vi "Init Load Cell DaqChannel.vi"(0 "task in":refnum<k21>, 1 "LoadCellParams":T2={"Excitation Value (Volts)"=2.5, "mV/V"=2.0, "Max Weight (lbs)"=500.0}, 2 "Do Offset Null?":bool, 5 "Physical Channels":tag, 7 "number samples":i32=1000, 9 "Rate":dbl=25000.0, 11 "error in (no error)":errorcluster, 12 "ShuntCalParams":T1={"Load Cell bridge resistance (Ohms)"=120.0, "9237 Internal shunt resistance (Ohms)"=100000.0, "shunt element location"=14813} {"shunt element location" items=["R1"=12465, "R2"=12466, "R3"=12467, "R4"=14813, "None"=10230]; "9237 Internal shunt resistance (Ohms)" format="%#.3p"}, 13 "Do Shunt Cal?":bool) -> (4 "task out":refnum<k21>, 15 "error out":errorcluster)   [LabVIEW 2017]
uses:
  <vilib>/DAQmx/create/scale.llb/DAQmx Create Scale (Linear).vi
  <vilib>/DAQmx/create/channels.llb/DAQmx Create Channel (AI-Voltage-Custom with Excitation).vi
  <vilib>/DAQmx/configure/timing.llb/DAQmx Timing (Sample Clock).vi
  <userlib>/_OpenG.lib/error/error.llb/Filter Error Codes (Array)__ogtk.vi
  <vilib>/DAQmx/calibration/calibrationInfo.llb/DAQmx Perform Shunt Calibration Ex (Bridge).vi
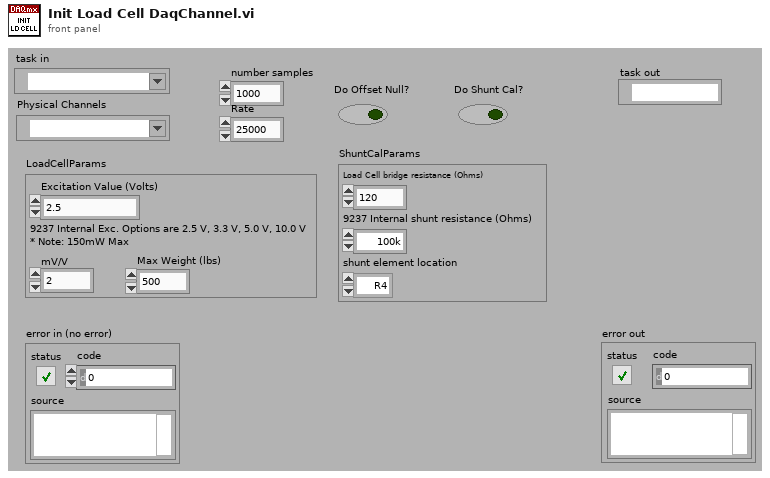
[diagram p1: front panel]
types:
  T1 = cluster{"Load Cell bridge resistance (Ohms)":dbl, "9237 Internal shunt resistance (Ohms)":dbl, "shunt element location":i32}
  T2 = cluster{"Excitation Value (Volts)":dbl, "mV/V":dbl, "Max Weight (lbs)":dbl}
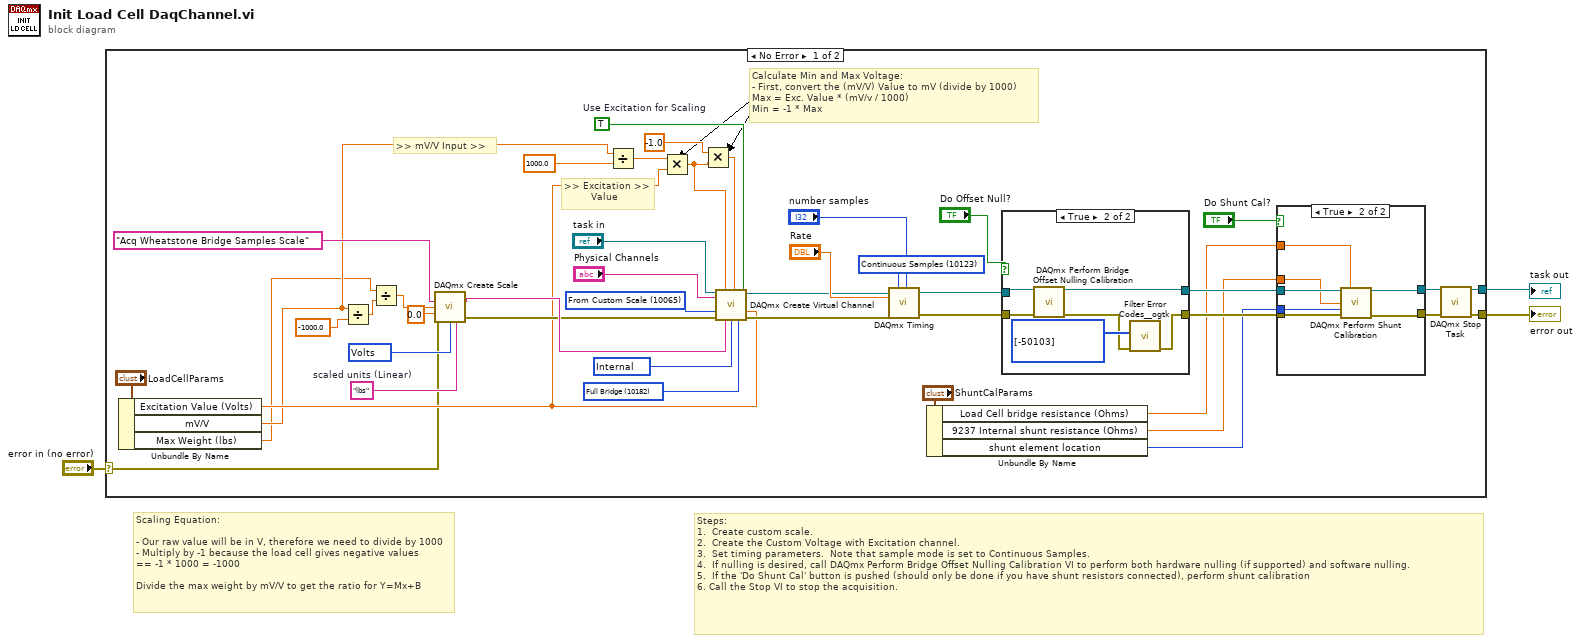
[diagram p0: block diagram]
diagram:
  # "Scaling Equation:\n\n- Our raw value will be in V, therefore we need to divide by 1000\n- Multiply by -1 because the load cell gives negative values\n== -1 * 1000 = -1000\n\nDivide the max weight by mV/V to get the ratio for Y=Mx+B"
  # "Steps:\n1.  Create custom scale.\n2.  Create the Custom Voltage with Excitation channel.\n3.  Set timing parameters.  Note that sample mode is set to Continuous Samples.\n4.  If nulling is desired, call DAQmx Perform Bridge Offset Nulling Calibration VI to perform both hardware nulling (if supported) and software nulling.\n5.  If the 'Do Shunt Cal' button is pushed (should only be done if you have shunt resistors connected), perform shunt calibration \n6. Call the Stop VI to stop the acquisition."
  n1 = case shown="No Error" "error in (no error)" {
    selector: "error in (no error)" -> [w5 w65]
    tunnel: [w18 w65] -> w3
    tunnel: [w16 _] -> w2
    frame No Error {
      w33 = "lbs"  # scaled units (Linear)
      w29 = 10348 items=["Volts"=10348, "Amps"=10342, "Deg F"=10144, "Deg C"=10143, "Deg R"=10145, "Kelvins"=10325, "Strain"=10299, "Ohms"=10384, "Hz"=10373, "Seconds"=10364] ("pre-scaled units")
      w36 = 10200 items=["Internal"=10200, "External"=10167, "None"=10230] ("Excitation Source")
      w35 = 10182 items=["Full Bridge"=10182, "Half Bridge"=10187, "Quarter Bridge"=10270, "No Bridge"=10228] ("Bridge Configuration")
      w30 = TRUE  # Use Excitation for Scaling
      w37 = 10065 items=["Volts"=10348, "From Custom Scale"=10065] ("units")
      w47 = 10123 items=["Finite Samples"=10178, "Continuous Samples"=10123] ("sample mode")
      # ">> Excitation >>\n         Value"
      # ">> mV/V Input >>"
      # "Calculate Min and Max Voltage:\n- First, convert the (mV/V) Value to mV (divide by 1000)\nMax = Exc. Value * (mV/v / 1000)\nMin = -1 * Max"
      n2 = Unbundle By Name("LoadCellParams") -> ("Excitation Value (Volts)"=w13:dbl, "mV/V"=w12:dbl, "Max Weight (lbs)"=w11:dbl)
      n3 = Divide(x=w12, y=-1000.0) -> (x/y=w23:dbl)
      n4 = Divide(x=w11, y=w23) -> (x/y=w20:dbl)
      n5 = call-poly <vilib>:"DAQmx Create Scale.vi"("name"="Acq Wheatstone Bridge Samples Scale", "slope"=w20, "y-intercept"=0.0 ("B"), "error in"=w5, "pre-scaled units"=w29, "scaled units"=w33) -> ("scale out"=w40:tag, "error out"=w39:errorcluster)  [unwired: 8 in]
      n6 = Divide(x=w12, y=1000.0) -> (x/y=w25:dbl)
      n7 = Multiply(x=w25, y=w13) -> (x*y=w22:dbl)
      n8 = Multiply(x=-1.0, y=w22) -> (x*y=w21:dbl)
      n9 = call-poly <vilib>:"DAQmx Create Virtual Channel.vi"("task in"="task in", "maximum value"=w22, "minimum value"=w21, "physical channels"="Physical Channels", "use excitation for scaling"=w30, "units"=w37, "voltage excitation value"=w13, "error in"=w39, "custom scale name"=w40, "voltage excitation source"=w36, "bridge configuration"=w35) -> ("task out"=w32:refnum<k21>, "error out"=w31:errorcluster)  [unwired: 3 in]
      n10 = call-poly <vilib>:"DAQmx Timing.vi"("task/channels in"=w32, "sample mode"=w47, "samples per channel"="number samples", "rate"="Rate", "error in"=w31) -> ("task out"=w42:refnum<k21>, "error out"=w41:errorcluster)  [unwired: 9 in]
      n11 = Unbundle By Name("ShuntCalParams") -> ("Load Cell bridge resistance (Ohms)"=w8:dbl, "9237 Internal shunt resistance (Ohms)"=w7:dbl, "shunt element location"=w6:i32)
      n12 = case shown="True" "Do Offset Null?" {
        tunnel: w42 -> [w49 w54]
        tunnel: w41 -> [w48 w53]
        tunnel: [w49 w55] -> w34
        tunnel: [w48 w50] -> w45
        frame False {
        }
        frame True {
          n13 = call <vilib>:"DAQmx Perform Bridge Offset Nulling Calibration.vi"("task/channels in"=w54, "error in"=w53) -> ("task out"=w55:refnum<k21>, "error out"=w51:errorcluster)  [unwired: 12 in]
          n14 = call-poly <userlib>:"Filter Error Codes__ogtk.vi"("Error In"=w51, "Error Codes to Filter"=i32[] [-50103]) -> ("Error Out"=w50:errorcluster)  [unwired: 7 in, 2 out]
        }
      }
      n15 = case shown="True" "Do Shunt Cal?" {
        tunnel: w34 -> [w56 w64]
        tunnel: w45 -> [w57 w62]
        tunnel: [w56 w63] -> w15
        tunnel: [w57 w61] -> w17
        tunnel: w8 -> [_ w60]
        tunnel: w7 -> [_ w59]
        tunnel: w6 -> [_ w58]
        frame False {
        }
        frame True {
          n16 = call-poly <vilib>:"DAQmx Perform Shunt Calibration.vi"("task/channels in"=w64, "bridge resistance"=w60, "shunt resistance"=w59, "shunt element location"=w58, "error in"=w62) -> ("task out"=w63:refnum<k21>, "error out"=w61:errorcluster)  [unwired: 9 in]
        }
      }
      n17 = call <vilib>:"DAQmx Stop Task.vi"("task/channels in"=w15, "error in"=w17) -> ("task out"=w16:refnum<k21>, "error out"=w18:errorcluster)  [unwired: 12 in]
    }
    frame Error {
    }
  }
  "task out" <- w2
  "error out" <- w3
